vi "VFH-read_file-watercalibforVNA.vi"(8 "error in":errorcluster, 10 "file path (dialog if empty)":path=path "C:/projects/Universitet/Master/code/data/1_Intial_measurements/cap.s1p") -> (0 "error out":errorcluster, 2 "output cluster":T1)   [LabVIEW 2020, in "VFH-VNA_File_Handler.lvlib"]
uses:
  VFH-VNA_File_Handler.lvlib
  VFH-file_cluster-NanoVNA.ctl
panel:
  out "string array 2":string[][](array[string])
  out "string array":string[](array[string])
  out "after substring":string
  out "text":string
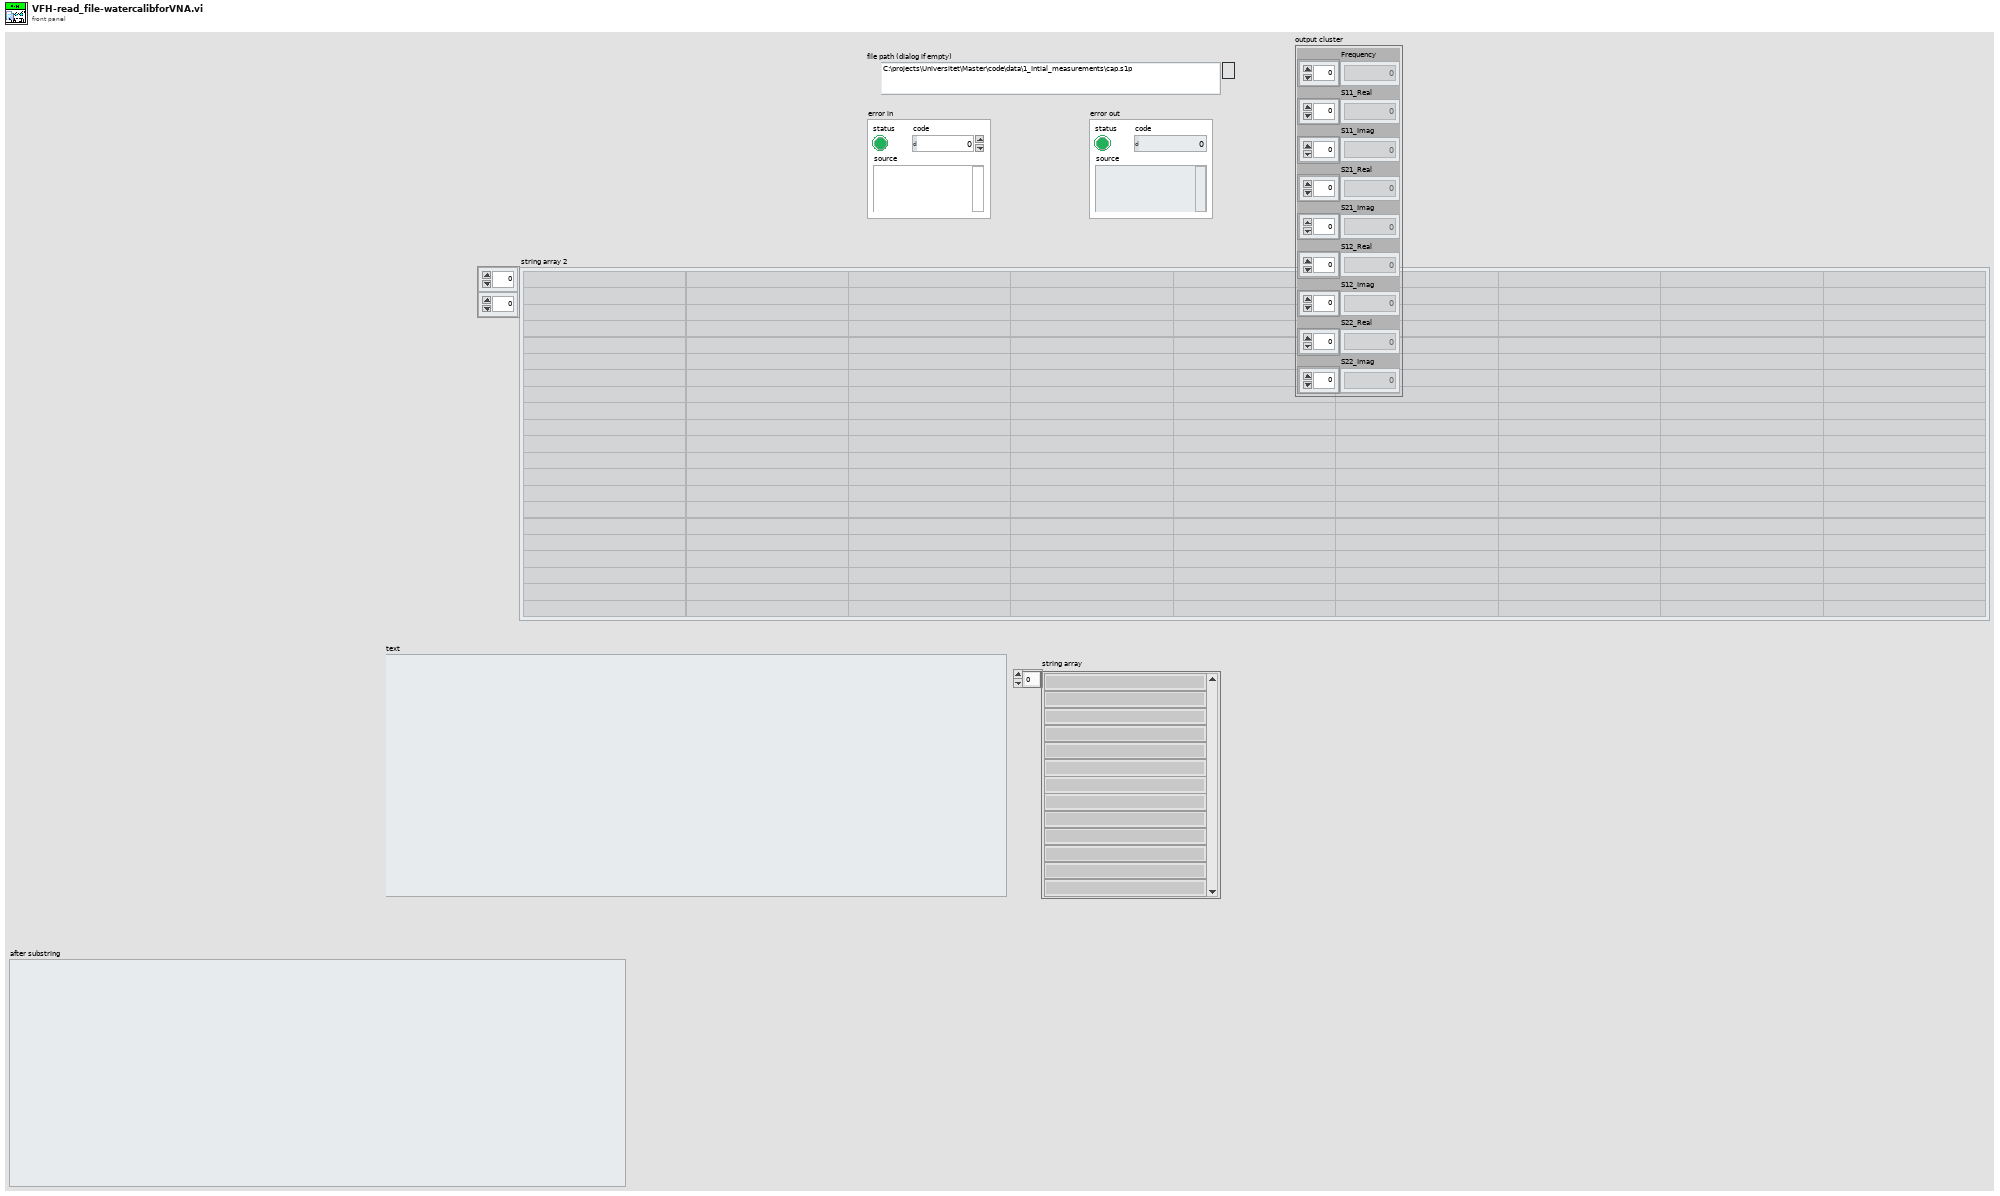
[diagram p1: front panel]
types:
  T1 = typedef "VFH-VNA_File_Handler.lvlib/VFH-file_cluster-NanoVNA.ctl" = cluster{"Frequency":dbl[], "S11_Real":dbl[], "S11_Imag":dbl[], "S21_Real":dbl[], "S21_Imag":dbl[], "S12_Real":dbl[], "S12_Imag":dbl[], "S22_Real":dbl[], "S22_Imag":dbl[]}
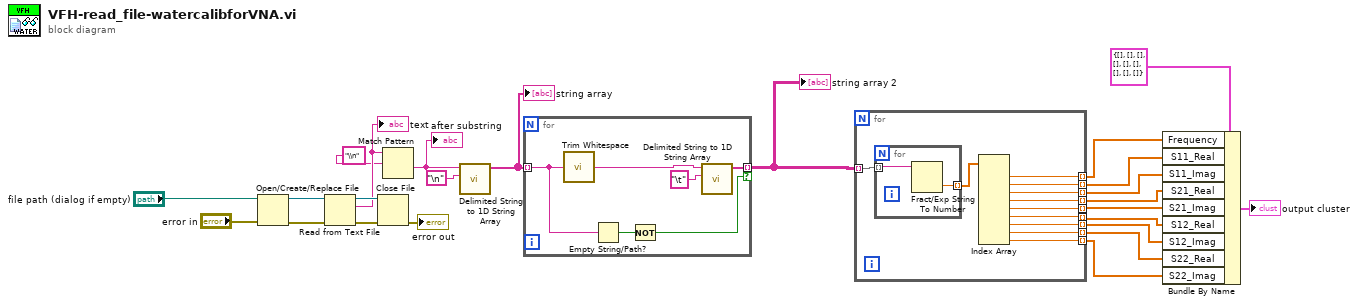
[diagram p0: block diagram]
diagram:
  n1 = Open/Create/Replace File(file path (use dialog)="file path (dialog if empty)", error in="error in") -> (refnum out=w24:refnum<file>, error out=w21:errorcluster)  [unwired: 4 in, 1 out]
  n2 = Read from Text File(file (use dialog)=w24, error in=w21) -> (refnum out=w23:refnum<file>, text=w19:string, error out=w22:errorcluster)  [unwired: 2 in, 1 out]
  "text" <- w19
  n3 = Close File(refnum=w23, error in=w22) -> (error out=→"error out":errorcluster)  [unwired: 1 out]
  n4 = Match Pattern(string=w19, regular expression="\\n" ("search string/char (-)")) -> (after substring=w15:string)  [unwired: 1 in, 3 out]
  "after substring" <- w15
  n5 = call <vilib>:"Delimited String to 1D String Array.vi"("delimiter"="\n", "delimited string"=w15) -> ("string array"=w16:string[])  [unwired: 9 in]
  "string array" <- w16
  n6 = for {
    tunnel: w16 -> [w26] mode=indexing
    tunnel: [w30] -> w14 mode=indexing if=w25
    n7 = call <vilib>:"Trim Whitespace.vi"("string"=w26) -> ("trimmed string"=w29:string)  [unwired: 1 in]
    n8 = Empty String/Path?(string/path=w26) -> (empty?=w27:bool)
    n9 = Not(x=w27) -> (.not. x?=w25:bool)
    n10 = call <vilib>:"Delimited String to 1D String Array.vi"("delimiter"="\t", "delimited string"=w29) -> ("string array"=w30:string[])  [unwired: 9 in]
  }
  "string array 2" <- w14
  n11 = for {
    tunnel: w14 -> [w41] mode=indexing
    tunnel: [w39] -> w13 mode=indexing
    tunnel: [w38] -> w12 mode=indexing
    tunnel: [w37] -> w11 mode=indexing
    tunnel: [w36] -> w10 mode=indexing
    tunnel: [w35] -> w9 mode=indexing
    tunnel: [w34] -> w8 mode=indexing
    tunnel: [w33] -> w7 mode=indexing
    tunnel: [w32] -> w6 mode=indexing
    tunnel: [w31] -> w5 mode=indexing
    n12 = for {
      tunnel: w41 -> [w43] mode=indexing
      tunnel: [w42] -> w40 mode=indexing
      n13 = Fract/Exp String To Number(string=w43) -> (number=w42:dbl)  [unwired: 3 in, 1 out]
    }
    n14 = Index Array(array=w40) -> (element #1=w39:dbl, element #2=w38:dbl, element #3=w37:dbl, element #4=w36:dbl, element #5=w35:dbl, element #6=w34:dbl, element #7=w33:dbl, element #8=w32:dbl, element #9=w31:dbl)  [unwired: 9 in]
  }
  n15 = Bundle By Name(cluster=T1 {"Frequency"=[], "S11_Real"=[], "S11_Imag"=[], "S21_Real"=[], "S21_Imag"=[], "S12_Real"=[], "S12_Imag"=[], "S22_Real"=[], "S22_Imag"=[]} ("output cluster"), "Frequency"=w13, "S11_Real"=w12, "S11_Imag"=w11, "S21_Real"=w10, "S21_Imag"=w9, "S12_Real"=w8, "S12_Imag"=w7, "S22_Real"=w6, "S22_Imag"=w5) -> (→"output cluster":T1)
